vi "Untitled 8.vi"() -> ()   [LabVIEW 2015]
uses:
  Controls/Sample Transfer Container Enumerator.ctl
  Controls/Sample Transfer Control Enumerator.ctl
  <vilib>/NIScanEngine/faults/Fault.ctl
panel:
  out "data":errorcluster
  out "Boolean array 2":bool[](array[boolean])
  out "x/y":dbl
  out "x = y?":bool
  in  "Sample Transfer Control":T1
  out "Boolean array":bool[](array[boolean])
  in  "Container 2":T2
  in  "Container":T2
  in  "Open/Close":bool
  out "Array 3":bool[](array[boolean])
  in  "Array 2":bool[](array[boolean])
  in  "Array":bool[](array[boolean])
  out "x .implies. y?":bool
  in  "ONOFF":bool
  in  "x":bool
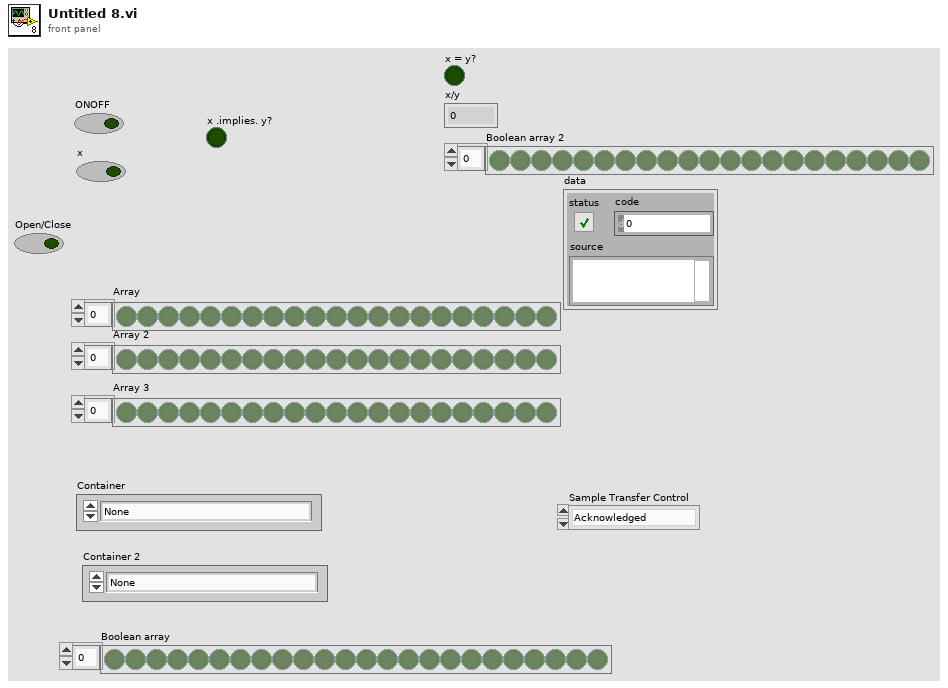
[diagram p1: front panel]
types:
  T1 = typedef "Sample Transfer Control Enumerator.ctl" = enum16{"Acknowledged", "Transfer", "Stash", "Abort", "Reset to Idle"}
  T2 = typedef "Sample Transfer Container Enumerator.ctl" = enum16{"None", "Sample 1", "Sample 2", "Sample 3", "Sample 4", "Sample 5", "Storage 01", "Storage 02", "Storage 03", "Storage 04", "Storage 05", "Storage 06", "Storage 07", "Storage 08", "Storage 09", "Storage 10", "Storage 11", "Storage 12", "Syringe", "Undefined"}
  T3 = typedef "Fault.ctl" = cluster{"code":i32, "level":i32, "first reported time":timestamp, "number reported":u32}
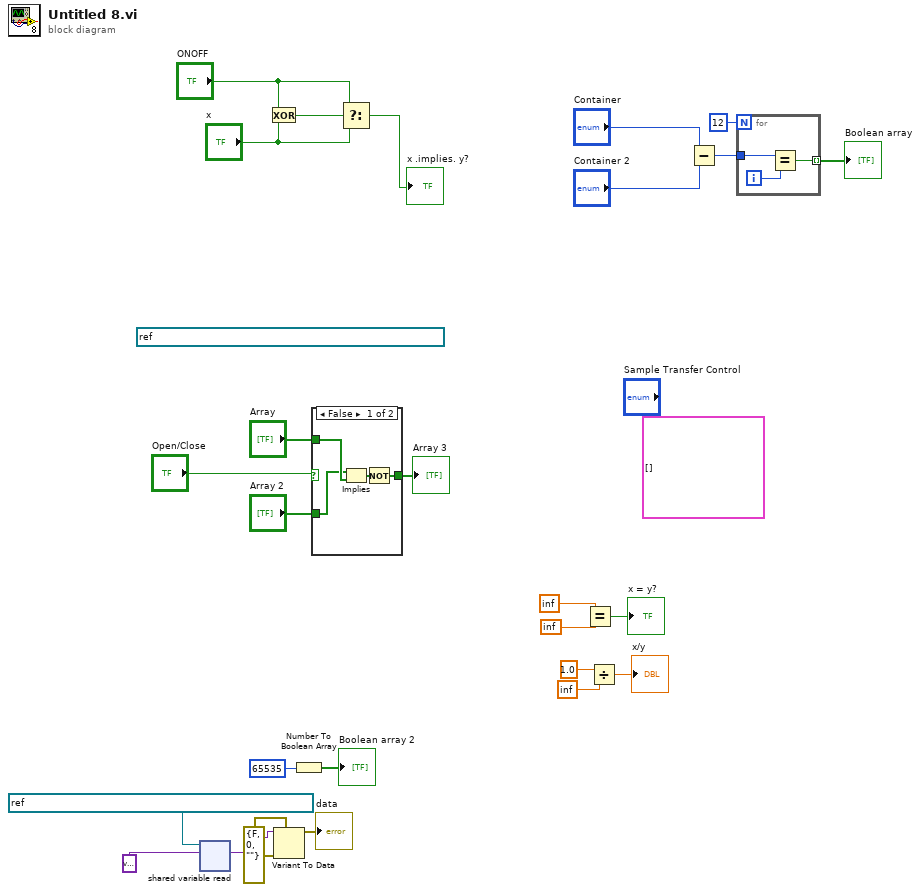
[diagram p0: block diagram]
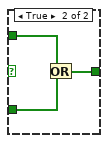
[diagram p2: hidden frame]
diagram:
  w2 = errorcluster {"status"=FALSE, "code"=0, "source"=""} ("error in")
  (unwired) T3[] [] ("fault list")
  (unwired) refnum<k21> "\\\\10.2.0.20\\NI_SystemState\\ControllerStatus\\FaultList"
  n1 = shared-variable-read(refnum<k21> "ni.var.psp://10.2.0.20/AMS Gas SHV/Outer Core Error" ("shared variable refnum in"), variant) -> (w3:variant)  [unwired: 1 in, 3 out]
  n2 = Exclusive Or(1:"x", 2:"ONOFF") -> (0:w26:bool)
  n3 = Variant To Data(error in=w2, type=w2, Variant=w3) -> (data=→"data":errorcluster)  [unwired: 1 out]
  n4 = Number To Boolean Array(number=u16 65535 ("Bit Field")) -> (Boolean array=→"Boolean array 2":bool[])
  n5 = case shown="False" "Open/Close" {
    tunnel: "Array" -> [w30 w33]
    tunnel: "Array 2" -> [w29 w32]
    tunnel: [w27 w31] -> w20
    frame False {
      n6 = Implies(1:w30, 2:w29) -> (0:w28:bool[])
      n7 = Not(x=w28) -> (.not. x?=w27:bool[])
    }
    frame True {
      n8 = Or(x=w33, y=w32) -> (x .or. y?=w31:bool[])
    }
  }
  "Array 3" <- w20
  n9 = Select(t="ONOFF", s=w26, f="x") -> (s? t:f=→"x .implies. y?":bool)
  n10 = Equal?(x=inf, y=inf) -> (x = y?=→"x = y?":bool)
  n11 = Divide(x=1.0, y=inf) -> (x/y=→"x/y":dbl)
  n12 = Subtract(x="Container", y="Container 2") -> (x-y=w16:u16)
  n13 = for {
    N: 12 -> [_]
    tunnel: w16 -> [w36]
    tunnel: [w34] -> w15 mode=indexing
    i -> [w35]
    n14 = Equal?(x=w36, y=w35) -> (x = y?=w34:bool)
  }
  "Boolean array" <- w15
